vi "Practica3.2_Secuence stacket.vi"() -> ()   [LabVIEW 2022 SP3]
panel:
  out "A < B":bool
  out "A > B":bool
  out "A = B":bool
  out "Multiplica A x B":dbl
  out "Divide A/B":dbl
  out "Resta A - B":dbl
  out "Suma A + B":dbl
  in  "Variable B":dbl
  in  "Vaiable A":dbl
  # "Anahí Montserrat Vázquez Padilla \nPráctica 03: Secuence Staquet \n31/01/2024"
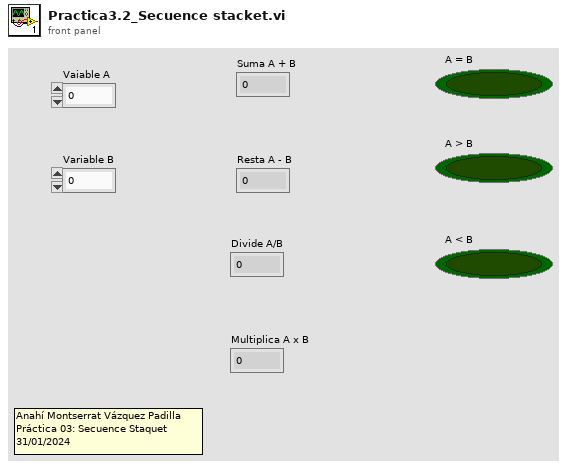
[diagram p1: front panel]
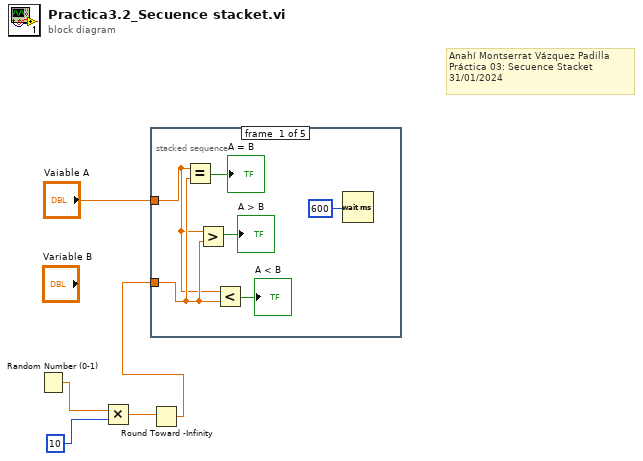
[diagram p0: block diagram]
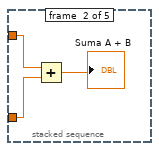
[diagram p2: hidden frame]
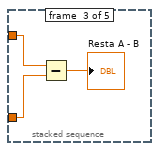
[diagram p3: hidden frame]
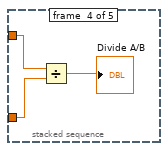
[diagram p4: hidden frame]
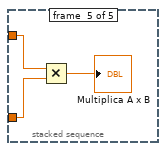
[diagram p5: hidden frame]
diagram:
  # "Anahí Montserrat Vázquez Padilla \nPráctica 03: Secuence Stacket \n31/01/2024"
  n1 = Random Number (0-1)() -> (number: 0 to 1=w4:dbl)
  n2 = Multiply(x=w4, y=10) -> (x*y=w2:dbl)
  n3 = Round Toward -Infinity(1:w2) -> (0:w1:dbl)
  n4 = stacked-sequence {
    tunnel: "Vaiable A" -> [w7 w14 w16 w19 w22]
    tunnel: w1 -> [w8 w13 w17 w20 w23]
    frame #0 {
      n5 = Equal?(x=w7, y=w8) -> (x = y?=→"A = B":bool)
      n6 = Greater?(x=w7, y=w8) -> (0:→"A > B":bool)
      n7 = Less?(x=w7, y=w8) -> (x < y?=→"A < B":bool)
      n8 = Wait (ms)(milliseconds to wait=600) -> ()  [unwired: 1 out]
    }
    frame #1 {
      n9 = Add(x=w14, y=w13) -> (x+y=→"Suma A + B":dbl)
    }
    frame #2 {
      n10 = Subtract(x=w16, y=w17) -> (x-y=→"Resta A - B":dbl)
    }
    frame #3 {
      n11 = Divide(x=w19, y=w20) -> (x/y=→"Divide A/B":dbl)
    }
    frame #4 {
      n12 = Multiply(x=w22, y=w23) -> (x*y=→"Multiplica A x B":dbl)
    }
  }
